vi "Simulate Acquired Data.vi"(8 "error in":errorcluster, 10 "Generated Data":string, 11 "Hardware Configuration in":T4) -> (0 "error out":errorcluster, 2 "Acquired Data":T13, 3 "Hardware Configuration out":T4)   [LabVIEW 2021, in "Acquisition.lvlib"]
doc: "Generate a separate waveform for each channel in 'Hardware Configuration in'."
uses:
  Acquisition.lvlib
  Acquired Data.ctl
  Hardware Configuration.ctl
  Channel Settings.ctl
  IO Device.ctl
  Sensor Type.ctl
  Interval Timer/Repeat Interval.ctl
  Interval Timer/Interval Length.ctl
  Interval Timer/Interval Token.ctl
  IO Context.ctl
  IO API.ctl
  Interval Timer/Interval Timer.lvlib
  Host Software Package.ctl
  Host IO Resource.ctl
  Host Resources.ctl
  support/Message Queue/Message Cluster.ctl
  support/Message Queue/Message Queue.lvlib
panel:
  in  "Diagnostics Queue":refnum<queue>
  in  "Host Resources":T1
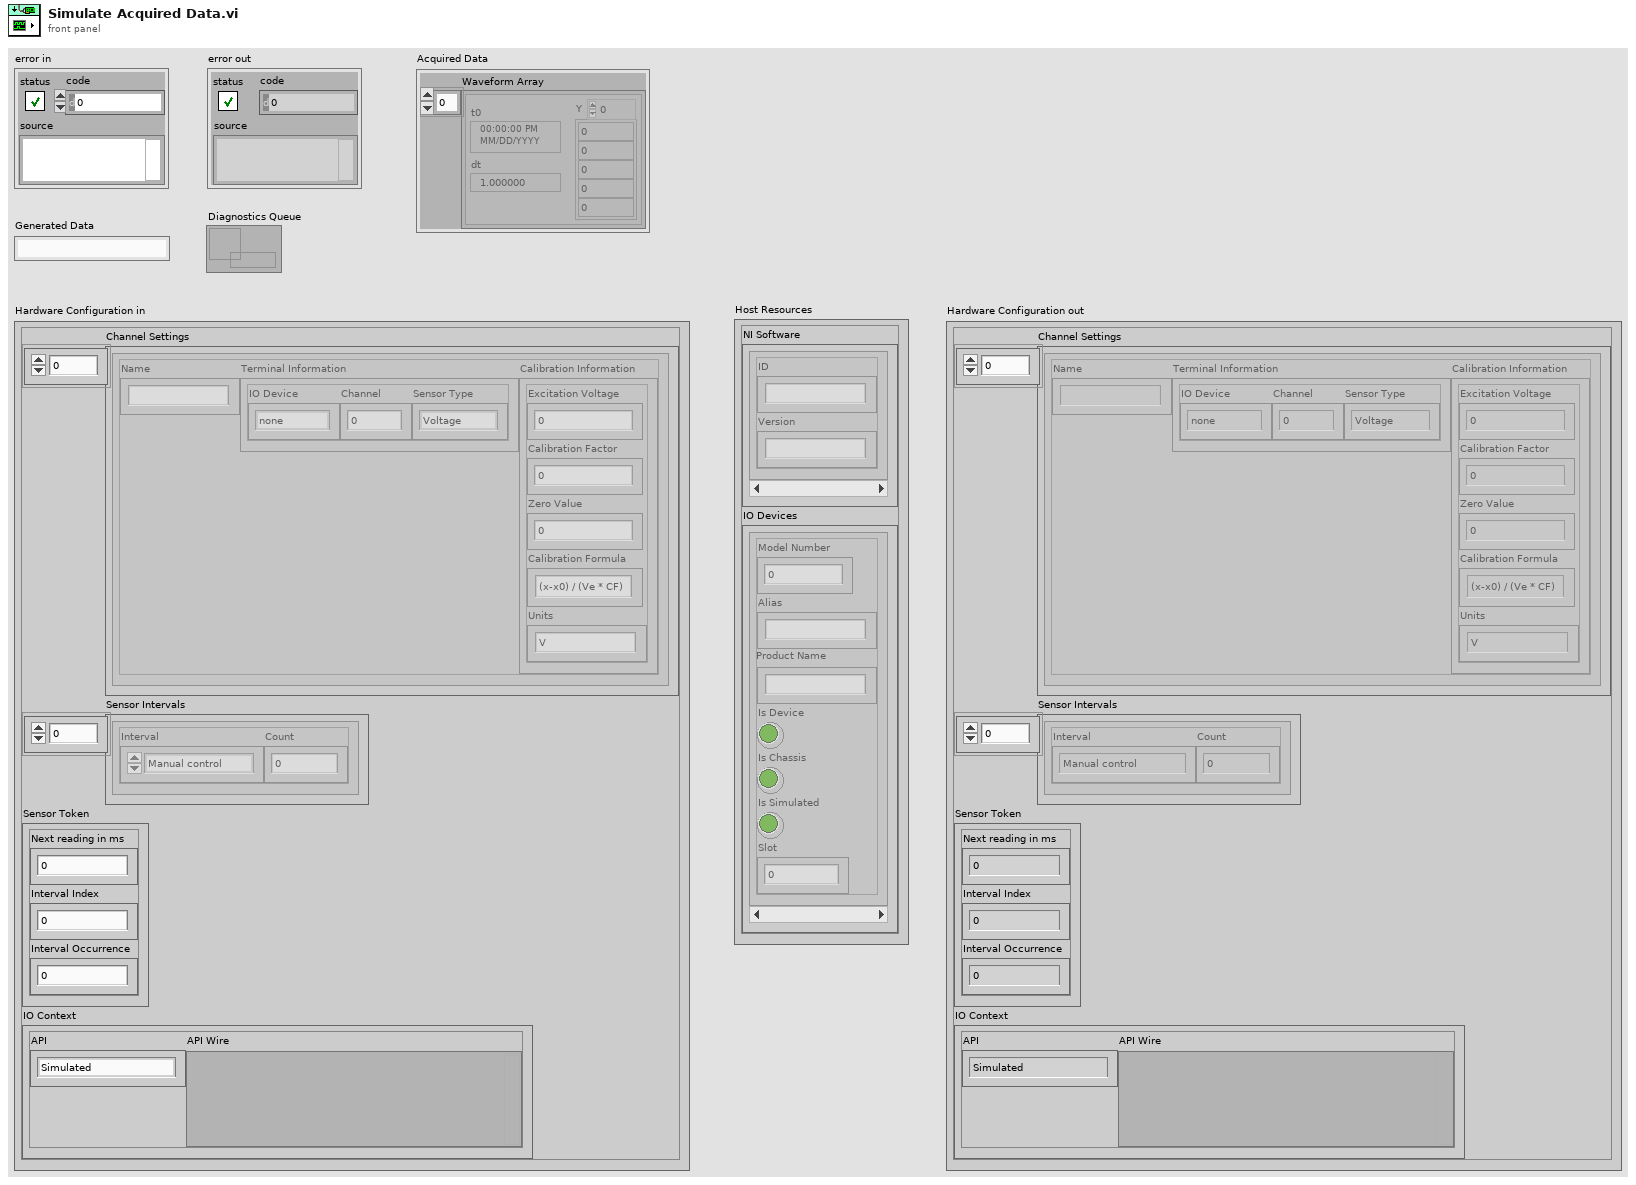
[diagram p1: front panel]
types:
  T1 = typedef "Acquisition.lvlib/Host Resources.ctl" = cluster{"NI Software":T2[], "IO Devices":T3[]}
  T2 = typedef "Acquisition.lvlib/Host Software Package.ctl" = cluster{"ID":string, "Version":string}
  T3 = typedef "Acquisition.lvlib/Host IO Resource.ctl" = cluster{"Model Number":u32, "Alias":string, "Product Name":string, "Is Device":bool, "Is Chassis":bool, "Is Simulated":bool, "Slot":i32}
  T4 = typedef "Acquisition.lvlib/Hardware Configuration.ctl" = cluster{"Channel Settings":T5[], "Sensor Intervals":T8[], "Sensor Token":T10, "IO Context":T11}
  T5 = typedef "Acquisition.lvlib/Channel Settings.ctl" = cluster{"Name":string, "Terminal Information":cluster{"IO Device":T6, "Channel":i32, "Sensor Type":T7}, "Calibration Information":cluster{"Excitation Voltage":dbl, "Calibration Factor":dbl, "Zero Value":dbl, "Calibration Formula":string, "Units":string}}
  T6 = typedef "Acquisition.lvlib/IO Device.ctl" = enum16{"none", "9219", "9401"}
  T7 = typedef "Acquisition.lvlib/Sensor Type.ctl" = enum16{"Voltage", "Load", "Pressure", "Encoder"}
  T8 = typedef "Interval Timer.lvlib/Repeat Interval.ctl" = cluster{"Interval":T9, "Count":i32}
  T9 = typedef "Interval Timer.lvlib/Interval Length.ctl" = enum16{"Manual control", "1 second", "10 seconds", "30 seconds", "60 seconds", "600 seconds", "1200 seconds", "3600 seconds"}
  T10 = typedef "Interval Timer.lvlib/Interval Token.ctl" = cluster{"Next reading in ms":u32, "Interval Index":i32, "Interval Occurrence":i32}
  T11 = typedef "Acquisition.lvlib/IO Context.ctl" = cluster{"API":T12, "API Wire":variant}
  T12 = typedef "Acquisition.lvlib/IO API.ctl" = enum16{"Simulated", "DAQmx"}
  T13 = typedef "Acquisition.lvlib/Acquired Data.ctl" = cluster{"Waveform Array":waveform(dbl)[]}
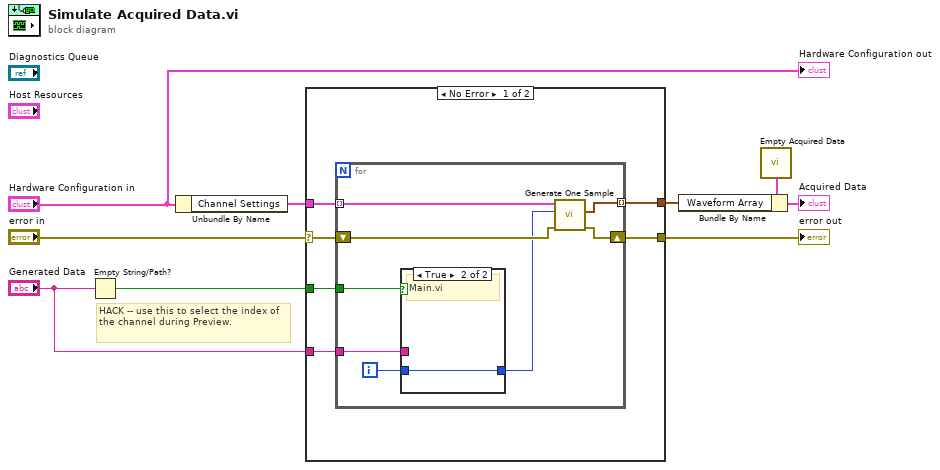
[diagram p0: block diagram]
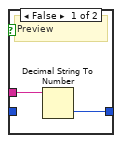
[diagram p2: hidden frame]
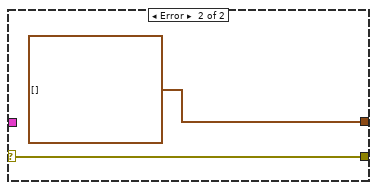
[diagram p3: hidden frame]
diagram:
  # "HACK -- use this to select the index of the channel during Preview."
  n1 = Empty String/Path?(string/path="Generated Data") -> (empty?=w2:bool)
  n2 = Unbundle By Name("Hardware Configuration in") -> ("Channel Settings"=w4:T5[])
  n3 = case shown="No Error" "error in" {
    selector: "error in" -> [w14 w28]
    tunnel: [w15 w28] -> w8
    tunnel: w4 -> [w13 _]
    tunnel: [w12 waveform(dbl)[] []] -> w6
    tunnel: w2 -> [w11 _]
    tunnel: "Generated Data" -> [w10 _]
    frame No Error {
      n4 = for {
        shift-right: [w23] -> w15
        shift-left: w14 -> [w21]
        tunnel: w13 -> [w22] mode=indexing
        tunnel: [w20] -> w12 mode=indexing
        tunnel: w11 -> [w19]
        tunnel: w10 -> [w16]
        i -> [w18]
        n5 = case shown="True" w19 {
          tunnel: w18 -> [_ w26]
          tunnel: [w24 w26] -> w17
          tunnel: w16 -> [w25 _]
          frame False {
            # "Preview"
            n6 = Decimal String To Number(string=w25) -> (number=w24:i32)  [unwired: 2 in, 1 out]
          }
          frame True {
            # "Main.vi"
          }
        }
        n7 = call "Generate One Sample.vi"("error in (no error)"=w21, "Active channel index"=w17, "Channel Settings"=w22) -> ("error out"=w23:errorcluster, "Waveform"=w20:waveform(dbl))  [unwired: 7 in]
      }
    }
    frame Error {
    }
  }
  "error out" <- w8
  n8 = call "Empty Acquired Data.vi"() -> ("Empty Acquired Data"=w5:T13)
  n9 = Bundle By Name(cluster=w5, "Waveform Array"=w6) -> (→"Acquired Data":T13)
  "Hardware Configuration out" <- "Hardware Configuration in"
